vi "ROSRegister.vi"(0 "Err In":string, 1 "ROS to register":T3={"topic port"=0, "Node"="", "topic"="", "type"="", "node port"=0, "error "={"status"=FALSE, "code"=0, "source"=""}, "Direction"=enum."Node", "APIs"=[], "Update (ms)"=1, "write queue"=1}) -> (2 "Err Out":string, 3 "Response":T2, 4 "MyState":T5, 5 "Log":T1)   [LabVIEW 2010]
uses:
  MyState.ctl
  _ROSDefinition.vi
  SubVIs/_ROSDirection.ctl
  SubVIs/_ROSControl.ctl
  ROSLog.ctl
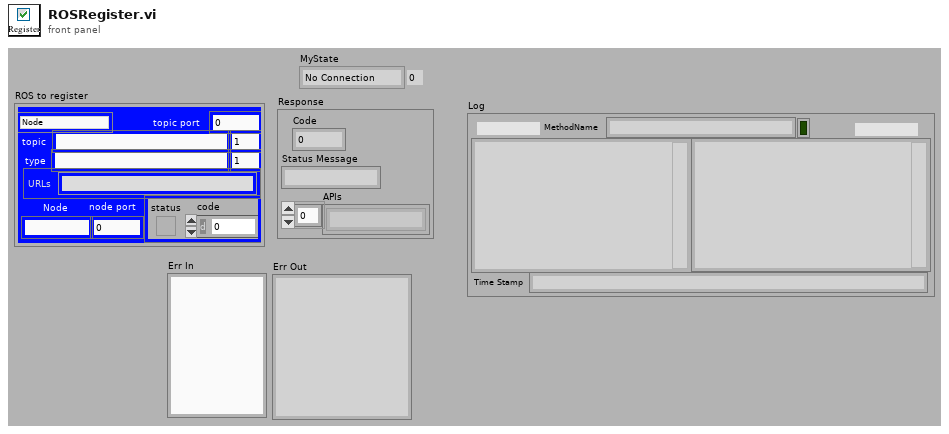
[diagram p1: front panel]
types:
  T1 = typedef "ROSLog.ctl" = cluster{"Sent":string, "Reply":string, "MethodName":string, "success":bool, "Dir1":string, "Dir2":string, "Time Stamp":string}
  T2 = cluster{"Code":i32, "Status Message":string, "APIs":string[]}
  T3 = typedef "_ROSControl.ctl" = cluster{"topic port":u16, "Node":string, "topic":string, "type":string, "node port":u32, "error ":errorcluster, "Direction":T4, "APIs":string[], "Update (ms)":u16, "write queue":u16}
  T4 = typedef "_ROSDirection.ctl" = enum16{"Node", "Publisher", "Subscriber", "Service Client"}
  T5 = typedef "MyState.ctl" = enum16{"No Connection", "Registered", "Connected", "Close"}
  T6 = enum16{"http://IP:port", "http://IP", "IP:port", "IP only"}
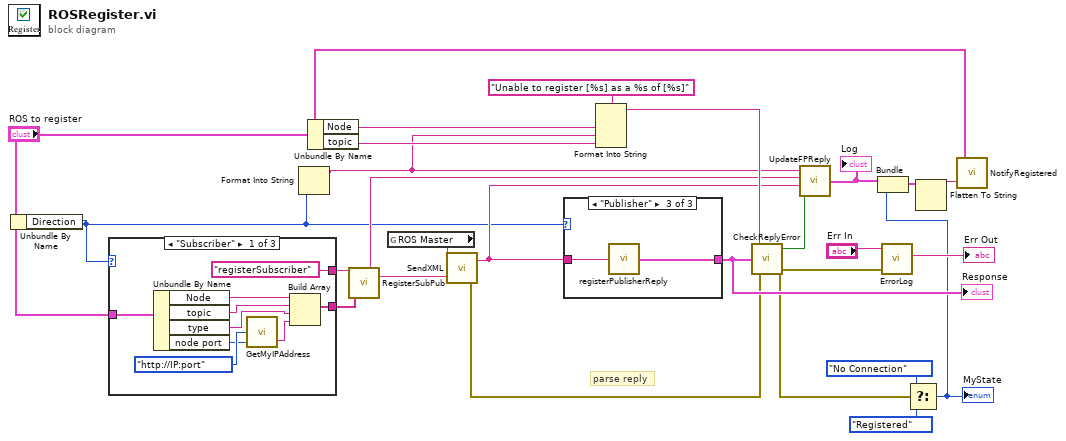
[diagram p0: block diagram]
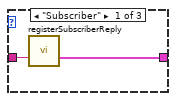
[diagram p2: hidden frame]
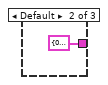
[diagram p3: hidden frame]
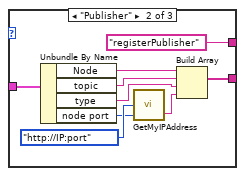
[diagram p4: hidden frame]
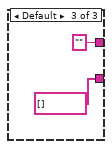
[diagram p5: hidden frame]
diagram:
  # "parse reply"
  n1 = Unbundle By Name("ROS to register") -> ("Direction"=w6:T4)
  n2 = case shown="\"Subscriber\"" w6 {
    tunnel: "ROS to register" -> [w28 w34 _]
    tunnel: ["registerSubscriber" ("MethodName") "registerPublisher" ("MethodName") "" ("MethodName")] -> w8
    tunnel: [w27 w35 string[] []] -> w7
    frame "Subscriber" {
      n3 = Unbundle By Name(w28) -> ("Node"=w32:string, "topic"=w31:string, "type"=w30:string, "node port"=w25:u32)
      n4 = call "GetMyIPAddress.vi"("Port"=w25, "Format"=T6."http://IP:port") -> ("URI"=w29:string)  [unwired: 2 in]
      n5 = Build Array(w32, w31, w30, w29) -> (w27:string[])
    }
    frame "Publisher" {
      n6 = Unbundle By Name(w34) -> ("Node"=w41:string, "topic"=w40:string, "type"=w39:string, "node port"=w38:u32)
      n7 = call "GetMyIPAddress.vi"("Port"=w38, "Format"=T6."http://IP:port") -> ("URI"=w37:string)  [unwired: 2 in]
      n8 = Build Array(w41, w40, w39, w37) -> (w35:string[])
    }
    frame Default {
    }
  }
  n9 = Format Into String(w6) -> (resulting string=w10:string)  [unwired: 3 in, 1 out]
  n10 = Unbundle By Name("ROS to register") -> ("Node"=w13:string, "topic"=w20:string)
  n11 = call "RegisterSubPub.vi"("Parameters"=w7, "MethodName"=w8) -> ("XML"=w9:string)
  n12 = global read "_ROSDefinition.vi" "ROS Master"() -> (w21:string)
  n13 = call "SendXML.vi"("Send"=w9, "URI in"=w21) -> ("error out"=w15:errorcluster, "Reply"=w11:string)
  n14 = case shown="\"Publisher\"" w6 {
    tunnel: [w45 T2 {"Code"=0, "Status Message"="", "APIs"=[]} ("Response") w49] -> w22
    tunnel: w11 -> [w46 _ w48]
    frame "Subscriber" {
      n15 = call "registerSubscriberReply.vi"("Response"=w46) -> ("Response"=w45:T2)
    }
    frame Default {
    }
    frame "Publisher" {
      n16 = call "registerPublisherReply.vi"("Response"=w48) -> ("Response"=w49:T2)
    }
  }
  "Response" <- w22
  n17 = Format Into String(format string="Unable to register [%s] as a %s of [%s]", w13, w10, w20) -> (resulting string=w14:string)  [unwired: 2 in, 1 out]
  n18 = call "CheckReplyError.vi"("error in"=w15, "Response"=w22, "Error String"=w14) -> ("error out"=w17:errorcluster, "Registered?"=w16:bool)  [unwired: 1 out]
  n19 = call "UpdateFPReply.vi"("success?"=w16, "Reply"=w11, "Sent"=w9, "method"=w10) -> ("Log"=w4:T1)
  "Log" <- w4
  n20 = call "ErrorLog.vi"("error in"=w17, "Error String"="Err In") -> ("String out"=→"Err Out":string)  [unwired: 1 in, 1 out]
  n21 = Select(t=MyState."No Connection" ("MyState"), s=w17, f=MyState."Registered" ("MyState")) -> (s? t:f=w3:T5)
  "MyState" <- w3
  n22 = Bundle("Log"=w4, "MyState"=w3) -> (w5:cluster{"Log":T1, "MyState":T5})  [unwired: 1 in]
  n23 = Flatten To String(anything=w5) -> (data string=w2:string)  [unwired: 3 in, 2 out]
  n24 = call "NotifyRegistered.vi"("data string"=w2, "ROS"="ROS to register") -> ()  [unwired: 2 in]
